vi "TER指令测试.vi"(2 "错误输入（无错误）":errorcluster, 3 "指令参数输入":T5={"测试指令1"={"写参数一"="+TXYBJT GPSQ", "写参数二"="+TXYBJT GPID", "读取版本号"="+TXYBJT GPST", "读取参数一"="+TXYBJT GPCH1", "读取参数二"="+TXYBJT GPCH2", "上电联网"="+TXYBJT GPSM", "指令下线"="+TXYBJT GPSS", "指示灯"=[]}, "测试指令2"={"读取信号强度"="+TXYBJT GPSQ", "读取SIM信息"="+TXYBJT GPID", "读取位置信息"="+TXYBJT GPST", "切换中心参数一"="+TXYBJT GPCH1", "切换中心参数二"="+TXYBJT GPCH2", "强制短信一"="+TXYBJT GPSM", "强制短信二"="+TXYBJT GPSS", "指示灯"=[]}, "等待时间"=[], "校验字符"=[], "GPRS参数"={"GPRS参数一"="", "GPRS参数二"=""}}, 4 "串口设置":T1={"COM号"="COM1", "波特率"=9600, "数据比特"=8, "奇偶"=enum."None", "停止位"=10, "流控制"=0} {"流控制" items=["无"=0, "XON/XOFF"=1, "RTS/CTS"=2, "DTR/DSR"=4]; "停止位" items=["1.0"=10, "1.5"=15, "2.0"=20]; "波特率" items=["75"=75, "110"=110, "134"=134, "150"=150, "300"=300, "600"=600, "1200"=1200, "1800"=1800, "2400"=2400, "4800"=4800, "7200"=7200, "9600"=9600, "14400"=14400, "19200"=19200, "28800"=28800, "38400"=38400, "56000"=56000, "57600"=57600, "115200"=115200, "128000"=128000, "230400"=230400]}) -> (0 "错误输出":errorcluster, 1 "指令参数输出":T5={"测试指令1"={"写参数一"="+TXYBJT GPSQ", "写参数二"="+TXYBJT GPID", "读取版本号"="+TXYBJT GPST", "读取参数一"="+TXYBJT GPCH1", "读取参数二"="+TXYBJT GPCH2", "上电联网"="+TXYBJT GPSM", "指令下线"="+TXYBJT GPSS", "指示灯"=[]}, "测试指令2"={"读取信号强度"="+TXYBJT GPSQ", "读取SIM信息"="+TXYBJT GPID", "读取位置信息"="+TXYBJT GPST", "切换中心参数一"="+TXYBJT GPCH1", "切换中心参数二"="+TXYBJT GPCH2", "强制短信一"="+TXYBJT GPSM", "强制短信二"="+TXYBJT GPSS", "指示灯"=[]}, "等待时间"=[], "校验字符"=[], "GPRS参数"={"GPRS参数一"="", "GPRS参数二"=""}})   [LabVIEW 2015]
panel:
  out "当前串口设置":T1={"COM号"="", "波特率"=9600, "数据比特"=8, "奇偶"=enum."None", "停止位"=10, "流控制"=0} {"流控制" items=["无"=0, "XON/XOFF"=1, "RTS/CTS"=2, "DTR/DSR"=4]; "停止位" items=["1.0"=10, "1.5"=15, "2.0"=20]; "数据比特" min=5 max=8 step=1; "波特率" items=["75"=75, "110"=110, "134"=134, "150"=150, "300"=300, "600"=600, "1200"=1200, "1800"=1800, "2400"=2400, "4800"=4800, "7200"=7200, "9600"=9600, "14400"=14400, "19200"=19200, "28800"=28800, "38400"=38400, "56000"=56000, "57600"=57600, "115200"=115200, "128000"=128000, "230400"=230400]}
  in  "通讯参数":T2={"写入缓冲区"="+TXYBJT TECH", "等待时间（毫秒）"=500, "搜索字符串/字符(-)"="Software,VERdowa_v"}
  out "测试指令2":T3={"读取信号强度"="+TXYBJT GPSQ", "读取SIM信息"="+TXYBJT GPID", "读取位置信息"="+TXYBJT GPST", "切换中心参数一"="+TXYBJT GPCH1", "切换中心参数二"="+TXYBJT GPCH2", "强制短信一"="+TXYBJT GPSM", "强制短信二"="+TXYBJT GPSS", "指示灯"=[]}
  out "测试指令1":T4={"写参数一"="+TXYBJT GPSQ", "写参数二"="+TXYBJT GPID", "读取版本号"="+TXYBJT GPST", "读取参数一"="+TXYBJT GPCH1", "读取参数二"="+TXYBJT GPCH2", "上电联网"="+TXYBJT GPSM", "指令下线"="+TXYBJT GPSS", "指示灯"=[]}
  in  "跳过按钮":bool
  out "动态显示数据":string
  out "暂存数据":string
  in  "输入数据":string
  # "TER   TCP  UDP  SMS"
  # "TER   TCP  UDP  SMS"
  # "TER   TCP  UDP  SMS"
  # "TER   TCP  UDP  SMS"
  # "TER   TCP  UDP  SMS"
  # "TER   TCP  UDP  SMS"
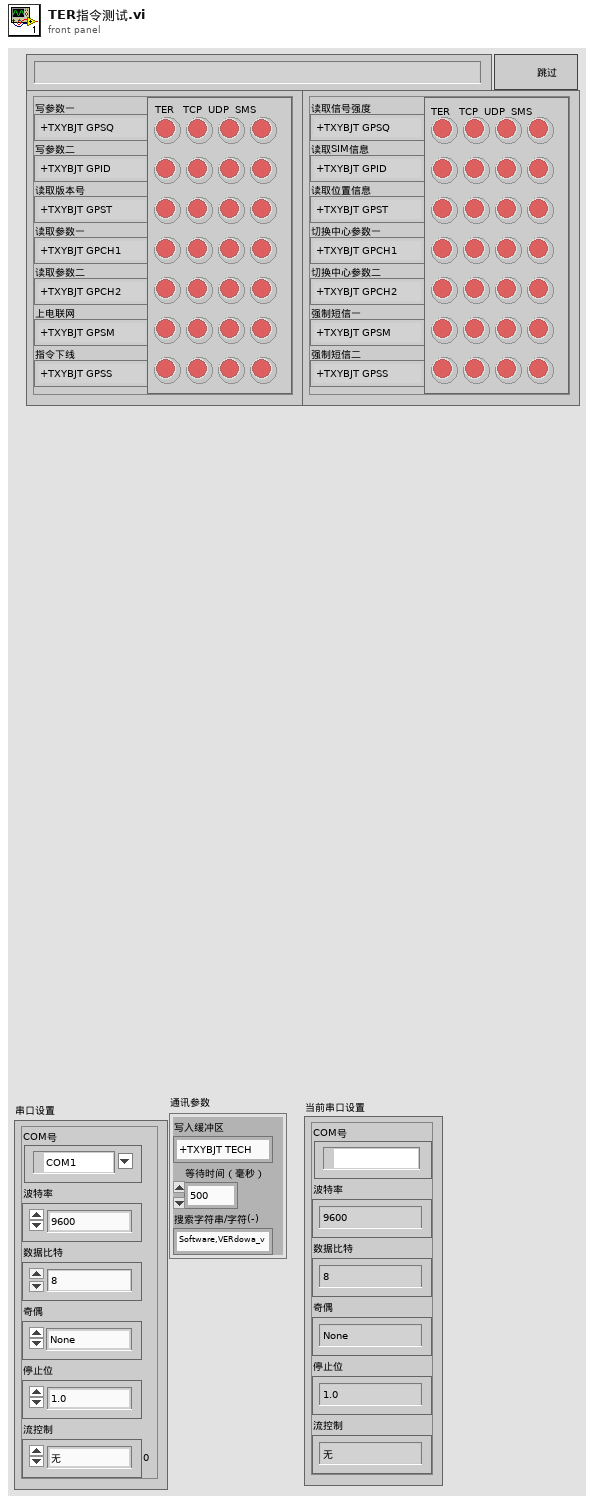
[diagram p1: front panel]
types:
  T1 = typedef "Serial - Settings.ctl" = cluster{"COM号":refnum<visa-resource-name>, "波特率":u32, "数据比特":u16, "奇偶":enum16{"None", "Odd", "Even", "Mark", "Space"}, "停止位":u16, "流控制":u16}
  T2 = cluster{"写入缓冲区":string, "等待时间（毫秒）":u32, "搜索字符串/字符(-)":string}
  T3 = typedef "指令参数2.ctl" = cluster{"读取信号强度":string, "读取SIM信息":string, "读取位置信息":string, "切换中心参数一":string, "切换中心参数二":string, "强制短信一":string, "强制短信二":string, "指示灯":bool[][]}
  T4 = cluster{"写参数一":string, "写参数二":string, "读取版本号":string, "读取参数一":string, "读取参数二":string, "上电联网":string, "指令下线":string, "指示灯":bool[][]}
  T5 = typedef "初始化测试指令.ctl" = cluster{"测试指令1":T6, "测试指令2":T3, "等待时间":u32[], "校验字符":string[], "GPRS参数":T7}
  T6 = typedef "指令参数1.ctl" = cluster{"写参数一":string, "写参数二":string, "读取版本号":string, "读取参数一":string, "读取参数二":string, "上电联网":string, "指令下线":string, "指示灯":bool[][]}
  T7 = typedef "GPRS参数.ctl" = cluster{"GPRS参数一":string, "GPRS参数二":string}
  T8 = typedef "TER状态机枚举.ctl" = enum16{"初始化", "等待按键", "显示", "写参数一", "写参数二", "退出"}
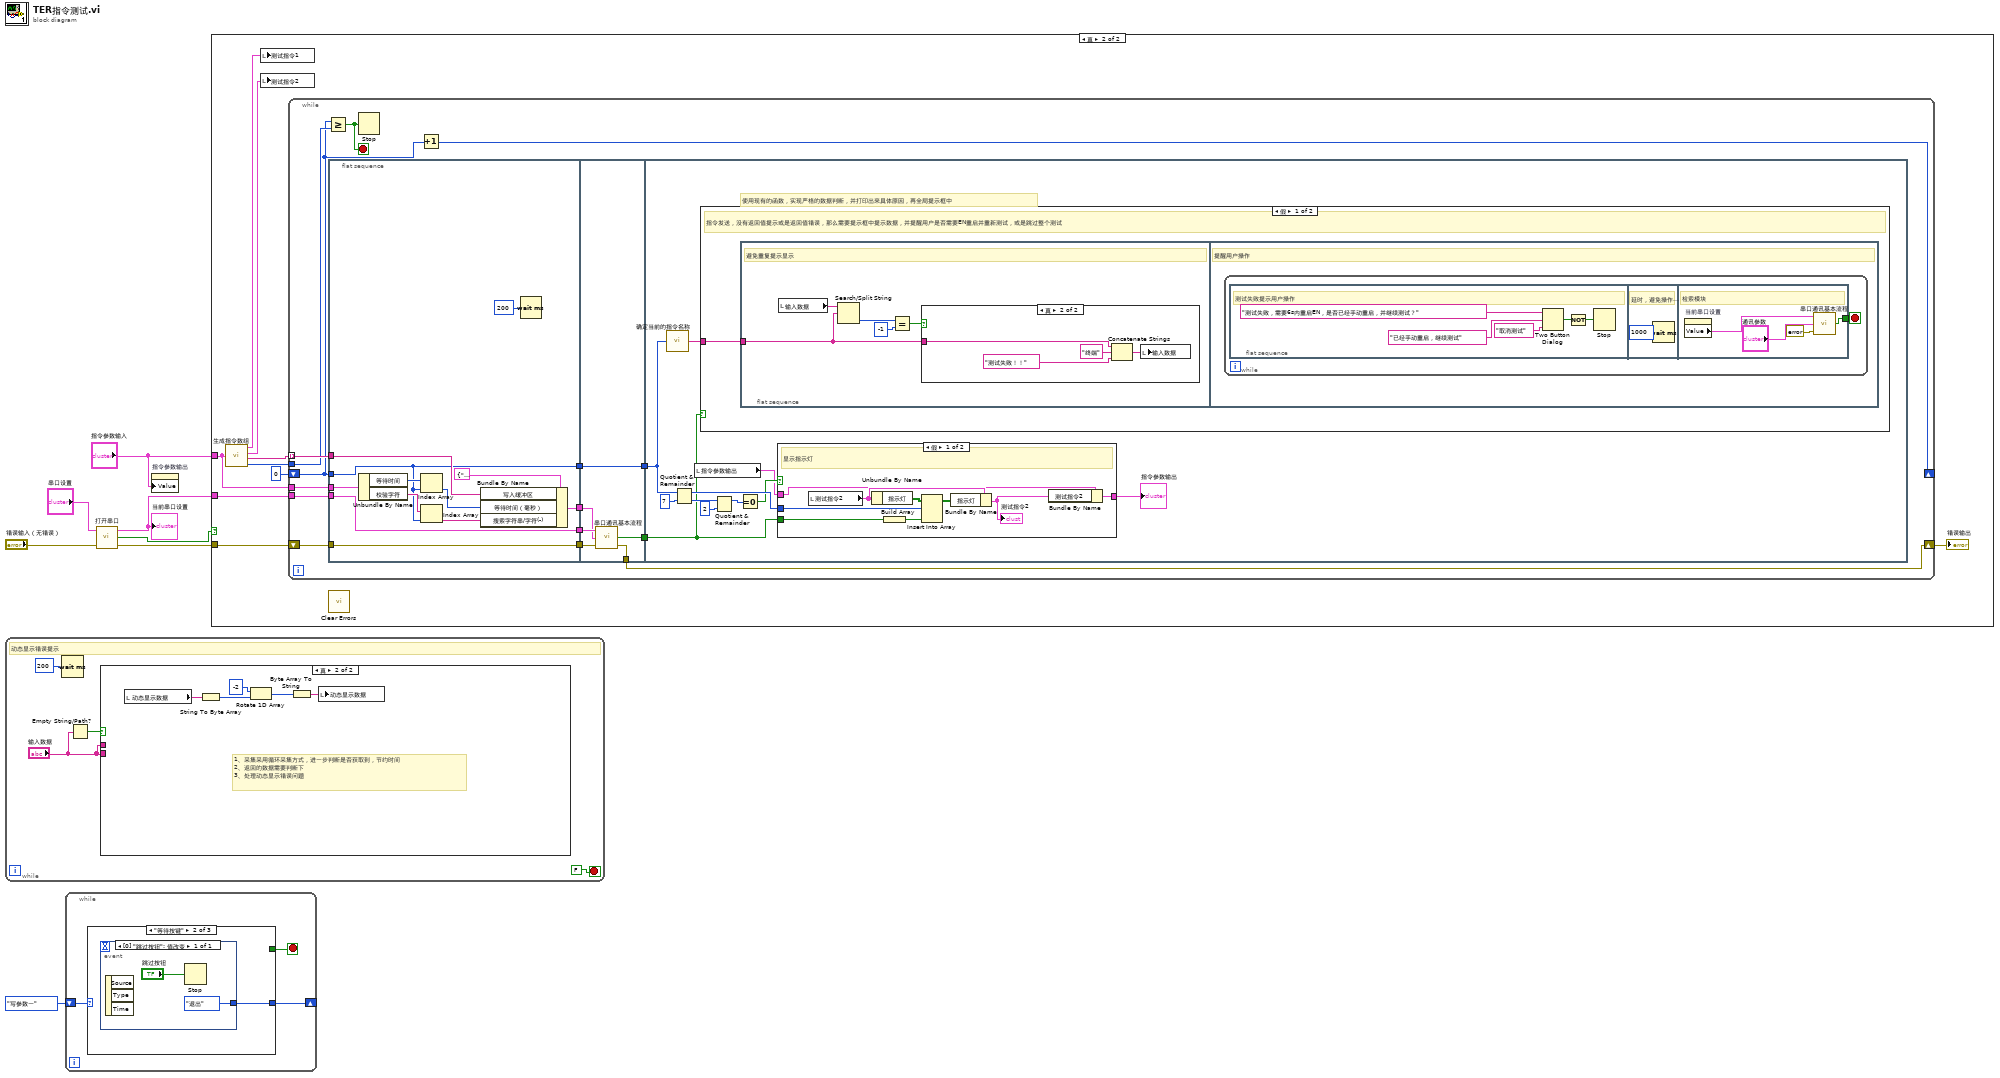
[diagram p0: block diagram]
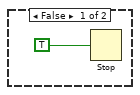
[diagram p2: hidden frame]
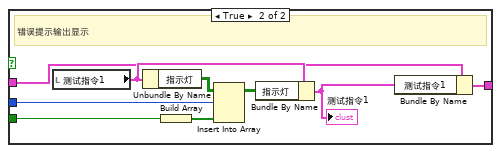
[diagram p5: hidden frame]
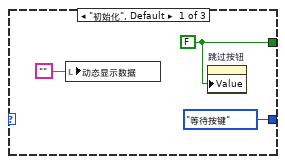
[diagram p6: hidden frame]
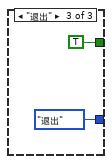
[diagram p7: hidden frame]
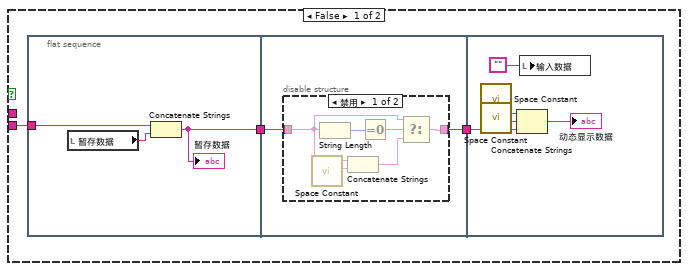
[diagram p8: hidden frame]
diagram:
  n1 = while {
    stop <- FALSE stop-if-true
    # "动态显示错误提示"
    n2 = Wait (ms)(milliseconds to wait=u32 200 ("等待时间（毫秒）")) -> ()  [unwired: 1 out]
    n3 = Empty String/Path?(string/path="输入数据") -> (empty?=w10:bool)
    n4 = case shown="真" w10 {
      tunnel: "输入数据" -> [w14 _]
      tunnel: "输入数据" -> [_ _]
      frame False {
        n5 = flat-sequence {
          tunnel: w14 -> [w15]
          tunnel: [w17] -> w13
          tunnel: w13 -> [w18]
          tunnel: [w19] -> w12
          tunnel: w12 -> [w31]
          frame #0 {
            n6 = local read "暂存数据"() -> (w16:string)
            n7 = Concatenate Strings(w15, w16) -> (w17:string)
            "暂存数据" <- w17
          }
          frame #1 {
            n8 = disable-structure shown="禁用" {
              disable-tunnel: [w23 w26] -> w19
              disable-tunnel: w18 -> [w22 w26]
              frame Disabled {
                n9 = call <vilib>:"Space Constant.vi"() -> ("String"=w20:string)
                n10 = String Length(string=w22) -> (length=w25:i32)
                n11 = Concatenate Strings(w22, w20) -> (w21:string)
                n12 = Equal To 0?(x=w25) -> (x = 0?=w24:bool)
                n13 = Select(t=w22, s=w24, f=w21) -> (s? t:f=w23:string)
              }
              frame Enabled {
              }
            }
          }
          frame #2 {
            n14 = call <vilib>:"Space Constant.vi"() -> ("String"=w29:string)
            n15 = call <vilib>:"Space Constant.vi"() -> ("String"=w30:string)
            n16 = Concatenate Strings(w29, w30, w31) -> (→"动态显示数据":string)
            n17 = local write "输入数据"("") -> ()
          }
        }
      }
      frame True {
        # "1、采集采用循环采集方式，进一步判断是否获取到，节约时间\n2、返回的数据需要判断下\n3、处理动态显示错误问题"
        n18 = local read "动态显示数据"() -> (w32:string)
        n19 = String To Byte Array(string=w32) -> (unsigned byte array=w36:u8[])
        n20 = Rotate 1D Array(1:w36, 2:-2 ("n")) -> (0:w35:u8[])
        n21 = Byte Array To String(unsigned byte array=w35) -> (string=w33:string)
        n22 = local write "动态显示数据"(w33) -> ()
      }
    }
  }
  n23 = while {
    shift-right: [w38] -> _
    shift-left: TER状态机枚举."写参数一" -> [w39]
    stop <- w37 stop-if-true
    n24 = case shown="\"等待按键\"" w39 {
      tunnel: [TER状态机枚举."等待按键" w43 TER状态机枚举."退出"] -> w38
      tunnel: [w40 _ TRUE] -> w37
      frame "初始化", Default {
        w40 = FALSE ("跳过按钮")
        n25 = local write "动态显示数据"("") -> ()
        n26 = property on="跳过按钮" class="Bool (严格)"("Value"=w40) -> ()  [unwired: 2 in, 2 out]
      }
      frame "等待按键" {
        n27 = event shown="[0] \"跳过按钮\": 值改变" {
          selector: _ -> [_]
          dyn-events: _ -> [_]
          timeout: _ -> [_]
          tunnel: [TER状态机枚举."退出"] -> w43
          event "跳过按钮": Value Change {
            n28 = event-data() -> ()  [unwired: 1 in, 3 out]
            n29 = Stop(stop? (T)="跳过按钮") -> ()
          }
        }
      }
      frame "退出" {
      }
    }
  }
  n30 = call "打开串口.vi"("错误输入（无错误）"="错误输入（无错误）", "串口设置"="串口设置") -> ("错误输出"=w3:errorcluster, "OpenOK?"=w6:bool, "串口设置输出"=w1:T1)  [unwired: 1 in]
  "当前串口设置" <- w1
  n31 = property on="指令参数输出" class="Clust (严格)"("Value"="指令参数输入") -> ()  [unwired: 2 in, 2 out]
  n32 = case shown="真" w6 {
    tunnel: w1 -> [_ w49]
    tunnel: w3 -> [_ w52]
    tunnel: "指令参数输入" -> [_ w50]
    frame False {
      n33 = Stop(stop? (T)=TRUE ("停止？(T)")) -> ()
    }
    frame True {
      n34 = call "生成指令数组.vi"("指令参数输入"=w50) -> ("测试指令1"=w55:T6, "测试指令2"=w54:T3, "数组"=w56:string[], "数值"=w57:i32)
      n35 = local write "测试指令1"(w55) -> ()
      n36 = local write "测试指令2"(w54) -> ()
      n37 = while {
        tunnel: w56 -> [w72] mode=indexing
        tunnel: w57 -> [w71]
        tunnel: w50 -> [w63]
        shift-right: [w58] -> w53
        shift-left: w52 -> [w69]
        tunnel: w49 -> [w68]
        shift-right: [w67] -> _
        shift-left: 0 -> [w66]
        stop <- w70 stop-if-true
        # "检测串口中断事件"
        n38 = Greater Or Equal?(x=w66, y=w71) -> (x >= y?=w70:bool)
        n39 = flat-sequence {
          tunnel: w68 -> [w84]
          tunnel: w72 -> [w81]
          tunnel: w66 -> [w74]
          tunnel: w69 -> [w75]
          tunnel: [w84] -> w65
          tunnel: [w82] -> w64
          tunnel: w63 -> [w80]
          tunnel: [w75] -> w62
          tunnel: [w74] -> w61
          tunnel: w62 -> [w88]
          tunnel: w64 -> [w89]
          tunnel: w65 -> [w90]
          tunnel: w61 -> [w87]
          tunnel: [w87] -> w60
          tunnel: [w86] -> w59
          tunnel: [w85] -> w58
          tunnel: w60 -> [w92]
          tunnel: w59 -> [w91]
          frame #0 {
            n40 = Unbundle By Name(w80) -> ("等待时间"=w79:u32[], "校验字符"=w77:string[])
            n41 = Index Array(array=w79, index=w74) -> (element=w78:u32)
            n42 = Index Array(array=w77, index=w74) -> (element=w76:string)
            n43 = Bundle By Name(cluster=T2 {"写入缓冲区"="+TXYBJT TECH", "等待时间（毫秒）"=500, "搜索字符串/字符(-)"="Software,VERdowa_v"} ("通讯参数"), "写入缓冲区"=w81, "等待时间（毫秒）"=w78, "搜索字符串/字符(-)"=w76) -> (w82:T2)
            n44 = Wait (ms)(milliseconds to wait=u32 200 ("等待时间（毫秒）")) -> ()  [unwired: 1 out]
          }
          frame #1 {
            n45 = call "串口通讯基本流程.vi"("错误输入（无错误）"=w88, "通讯参数"=w89, "串口设置"=w90) -> ("错误输出"=w85:errorcluster, "GetRightData？"=w86:bool)  [unwired: 1 out]
          }
          frame #2 {
            # "使用现有的函数，实现严格的数据判断，并打印出来具体原因，再全局提示框中"
            n46 = call "确定当前的指令名称.vi"("索引"=w92) -> ("指令名称"=w93:string)
            n47 = Quotient & Remainder(x=w92, y=7) -> (x-y*floor(x/y)=w100:i32, floor(x/y)=w99:i32)
            n48 = local read "指令参数输出"() -> (w94:T5)
            n49 = case shown="假" w91 {
              tunnel: w93 -> [w102 _]
              frame False {
                # "指令发送，没有返回值提示或是返回值错误，那么需要提示框中提示数据，并提醒用户是否需要EN重启并重新测试，或是跳过整个测试"
                n50 = flat-sequence {
                  tunnel: w102 -> [w103]
                  frame #0 {
                    # "避免重复提示显示"
                    n51 = local read "输入数据"() -> (w107:string)
                    n52 = Search/Split String(string=w107, search string/char (-)=w103) -> (offset of match=w106:i32)  [unwired: 1 in, 2 out]
                    n53 = Equal?(x=w106, y=-1) -> (x = y?=w104:bool)
                    n54 = case shown="真" w104 {
                      tunnel: w103 -> [_ w108]
                      frame False {
                      }
                      frame True {
                        n55 = Concatenate Strings(w108, "终端" ("字符串"), "测试失败！！" ("字符串")) -> (w111:string)
                        n56 = local write "输入数据"(w111) -> ()
                      }
                    }
                  }
                  frame #1 {
                    # "提醒用户操作"
                    n57 = while {
                      stop <- w112 stop-if-true
                      n58 = flat-sequence {
                        tunnel: [w122] -> w112
                        frame #0 {
                          # "测试失败提示用户操作"
                          n59 = Two Button Dialog(message="测试失败，需要6s内重启EN，是否已经手动重启，并继续测试？" ("消息"), 1:"取消测试" ("F按钮名称（“取消”）"), 2:"已经手动重启，继续测试" ("T按钮名称（“确定”）")) -> (T button?=w117:bool)
                          n60 = Not(x=w117) -> (.not. x?=w116:bool)
                          n61 = Stop(stop? (T)=w116) -> ()
                        }
                        frame #1 {
                          # "延时，避免操作过快"
                          n62 = Wait (ms)(milliseconds to wait=u32 1000 ("等待时间（毫秒）")) -> ()  [unwired: 1 out]
                        }
                        frame #2 {
                          # "检索模块"
                          n63 = property on="当前串口设置" class="Clust (严格)"() -> ("Value"=w119:T1)  [unwired: 2 in, 2 out]
                          n64 = call "串口通讯基本流程.vi"("错误输入（无错误）"=errorcluster {"status"=FALSE, "code"=0, "source"=""}, "通讯参数"="通讯参数", "串口设置"=w119) -> ("GetRightData？"=w122:bool)  [unwired: 2 out]
                        }
                      }
                    }
                  }
                }
              }
              frame True {
              }
            }
            n65 = Quotient & Remainder(x=w99, y=2) -> (x-y*floor(x/y)=w96:i32)  [unwired: 1 out]
            n66 = Equal To 0?(x=w96) -> (x = 0?=w97:bool)
            n67 = case shown="假" w97 {
              tunnel: w91 -> [w129 w136]
              tunnel: w100 -> [w127 w137]
              tunnel: [w126 w135] -> w95
              tunnel: w94 -> [w123 w132]
              frame False {
                # "显示指示灯"
                n68 = local read "测试指令2"() -> (w124:T3)
                n69 = Unbundle By Name(w124) -> ("指示灯"=w131:bool[][])
                n70 = Build Array(w129) -> (w128:bool[])
                n71 = Insert Into Array(array=w131, index (row)=w127, new element=w128) -> (w130:bool[][])  [unwired: 1 in]
                n72 = Bundle By Name(cluster=w124, "指示灯"=w130) -> (w125:T3)
                "测试指令2" <- w125
                n73 = Bundle By Name(cluster=w123, "测试指令2"=w125) -> (w126:T5)
              }
              frame True {
                # "错误提示输出显示"
                n74 = local read "测试指令1"() -> (w134:T4)
                n75 = Unbundle By Name(w134) -> ("指示灯"=w139:bool[][])
                n76 = Build Array(w136) -> (w140:bool[])
                n77 = Insert Into Array(array=w139, index (row)=w137, new element=w140) -> (w138:bool[][])  [unwired: 1 in]
                n78 = Bundle By Name(cluster=w134, "指示灯"=w138) -> (w133:T4)
                "测试指令1" <- w133
                n79 = Bundle By Name(cluster=w132, "测试指令1"=w133) -> (w135:T5)
              }
            }
            "指令参数输出" <- w95
          }
        }
        n80 = Stop(stop? (T)=w70) -> ()
        n81 = Increment(x=w66) -> (x+1=w67:i32)
      }
      "错误输出" <- w53
      n82 = call <vilib>:"Clear Errors.vi"() -> ()  [unwired: 6 in, 2 out]
    }
  }
